vi "Get Heater.vi"(6 "Channel":i32, 8 "error in (no error)":errorcluster, 11 "Instrument.Cryostat in":refnum<class "Instrument.Cryostat.lvclass">) -> (0 "error out":errorcluster, 1 "Status":string, 2 "Current (A)":dbl, 3 "Instrument.Cryostat out":refnum<class "Instrument.Cryostat.lvclass">)   [LabVIEW 2019, in "Instrument.Cryostat.lvclass"]
uses:
  Instrument.Cryostat.lvclass
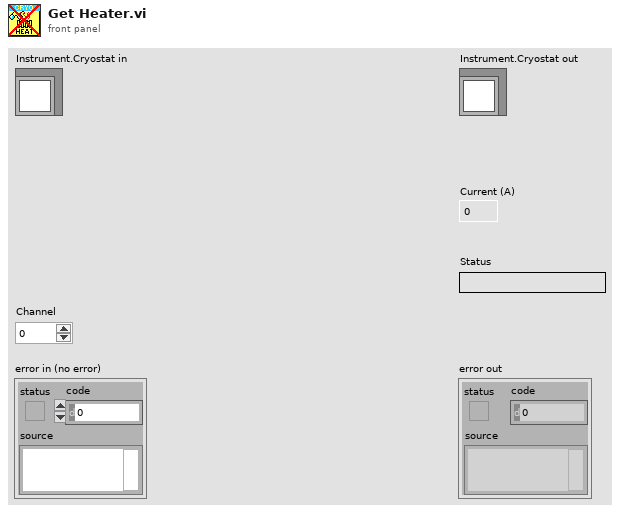
[diagram p1: front panel]
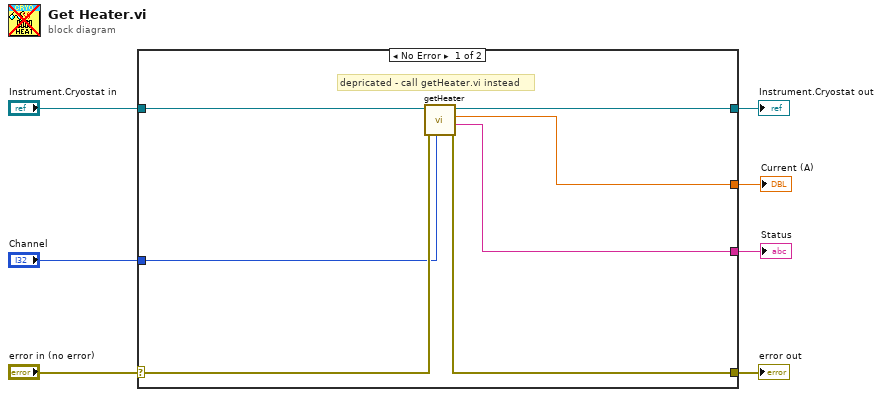
[diagram p0: block diagram]
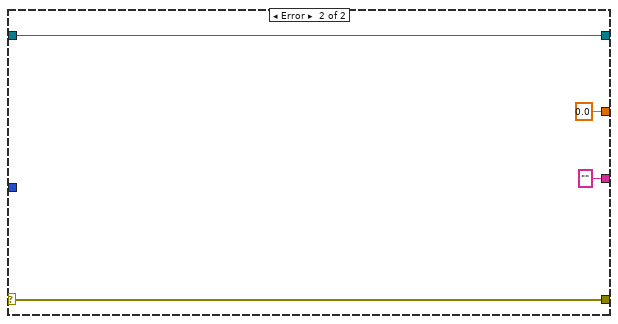
[diagram p2: hidden frame]
diagram:
  n1 = case shown="No Error" "error in (no error)" {
    selector: "error in (no error)" -> [w12 w18]
    tunnel: [w8 w18] -> w6
    tunnel: [w13 w17] -> w4
    tunnel: "Instrument.Cryostat in" -> [w14 w17]
    tunnel: "Channel" -> [w11 _]
    tunnel: [w10 "" ("Status")] -> w2
    tunnel: [w9 0.0 ("Current (A)")] -> w1
    frame No Error {
      # "depricated - call getHeater.vi instead"
      n2 = call-dynamic "getHeater.vi"("Channel"=w11, "error in (no error)"=w12, "Instrument.Cryostat in"=w14) -> ("error out"=w8:errorcluster, "Status"=w10:string, "Current (A)"=w9:dbl, "Instrument.Cryostat out"=w13:refnum<class "Instrument.Cryostat.lvclass">)  [unwired: 5 in]
    }
    frame Error {
    }
  }
  "error out" <- w6
  "Instrument.Cryostat out" <- w4
  "Current (A)" <- w1
  "Status" <- w2
